vi "Lookup MessageQs.vi"(7 "VolatusAPI":refnum<class "VolatusAPI.lvclass">, 8 "error in (no error)":errorcluster, 11 "LatchedValve in":refnum<class "LatchedValve.lvclass">) -> (0 "error out":errorcluster, 3 "LatchedValve out":refnum<class "LatchedValve.lvclass">)   [LabVIEW 2020, in "VolatusControl.lvlib" / "LatchedValve.lvclass"]
uses:
  LatchedValve.lvclass
  Volatus/VolatusAPI/VolatusAPI.lvclass
  LatchedValve.lvclass/LatchedValve.ctl
  Volatus/Module Identity/Module Identity.lvclass/Module Identity.ctl
  Volatus/Module Identity/Create.vi
  Volatus/Module Identity/Module Identity.lvclass
  C:/dev/lv20CE/relink/lv-volatus/Volatus/Identity/Identity.lvclass
  Volatus/VolatusAPI/Lookup Channel Info.vi
  Volatus/VolatusAPI/Lookup Q.vi
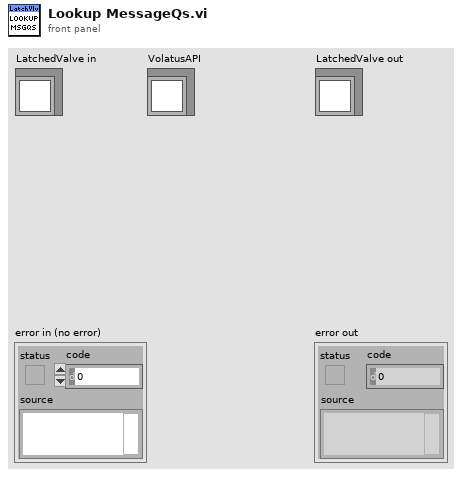
[diagram p1: front panel]
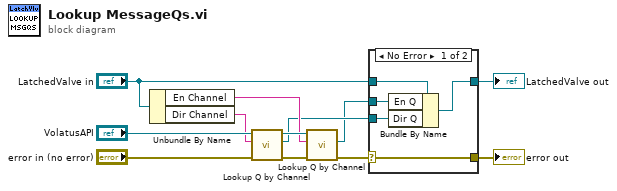
[diagram p0: block diagram]
diagram:
  n1 = Unbundle By Name("LatchedValve in") -> ("En Channel"=w3:string, "Dir Channel"=w5:string)
  n2 = call "Lookup Q by Channel.vi"("error in (no error)"="error in (no error)", "Channel Name"=w5, "VolatusAPI in"="VolatusAPI") -> ("error out"=w6:errorcluster, "MessageQ"=w2:refnum<class "MessageQ.lvclass">, "VolatusAPI out"=w4:refnum<class "VolatusAPI.lvclass">)  [unwired: 6 in]
  n3 = call "Lookup Q by Channel.vi"("error in (no error)"=w6, "Channel Name"=w3, "VolatusAPI in"=w4) -> ("error out"=w7:errorcluster, "MessageQ"=w1:refnum<class "MessageQ.lvclass">)  [unwired: 6 in, 1 out]
  n4 = case shown="No Error" w7 {
    selector: w7 -> [w13 w19]
    tunnel: "LatchedValve in" -> [w17 w18]
    tunnel: [w16 w18] -> w11
    tunnel: [w13 w19] -> w10
    tunnel: w2 -> [w15 _]
    tunnel: w1 -> [w14 _]
    frame No Error {
      n5 = Bundle By Name(cluster=w17, "En Q"=w14, "Dir Q"=w15) -> (w16:refnum<class "LatchedValve.lvclass">)
    }
    frame Error {
    }
  }
  "error out" <- w10
  "LatchedValve out" <- w11
